vi "Apply Density.vi"(0 "ToneCloud in":refnum<class "Tone Cloud.lvclass">, 11 "error in (no error)":errorcluster) -> (4 "ToneCloud out":refnum<class "Tone Cloud.lvclass">, 15 "error out":errorcluster)   [LabVIEW 2015, in "Tone Cloud.lvclass"]
uses:
  Tone Cloud.lvclass
  Tone Cloud.lvclass/Tone Cloud.ctl
  <vilib>/regexp/Match Regular Expression.xnode
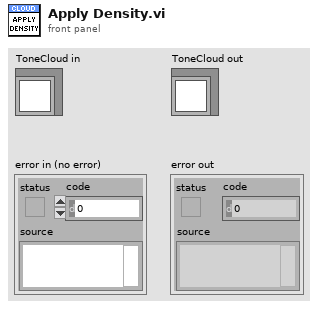
[diagram p1: front panel]
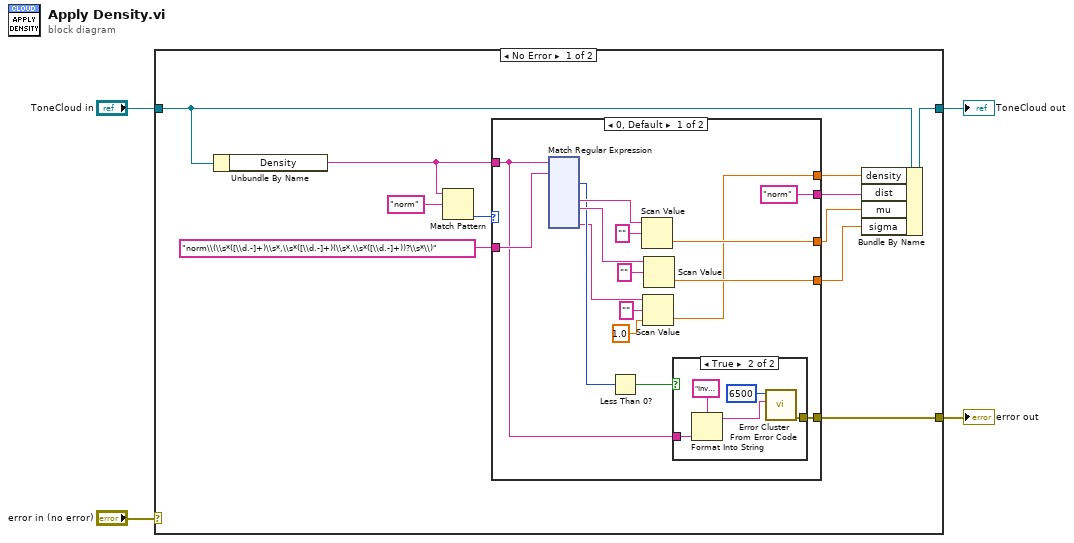
[diagram p0: block diagram]
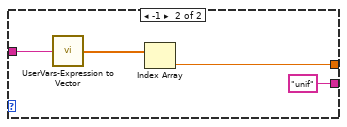
[diagram p3: hidden frame]
diagram:
  n1 = case shown="No Error" "error in (no error)" {
    selector: "error in (no error)" -> [_ w161]
    tunnel: [w5 w161] -> w3
    tunnel: [w14 w160] -> w1
    tunnel: "ToneCloud in" -> [w15 w160]
    frame No Error {
      n2 = Unbundle By Name(w15) -> ("Density"=w12:string)
      n3 = Match Pattern(string=w12, regular expression="norm") -> (offset past match=w10:i32)  [unwired: 1 in, 3 out]
      n4 = case shown="0, Default" w10 {
        tunnel: [w16 w158] -> w13
        tunnel: w12 -> [w21 w157]
        tunnel: ["norm" "unif"] -> w9
        tunnel: "norm\\(\\s*([\\d.-]+)\\s*,\\s*([\\d.-]+)(\\s*,\\s*([\\d.-]+))?\\s*\\)" ("String") -> [w30 _]
        tunnel: [w28 _] -> w7
        tunnel: [w24 _] -> w6
        tunnel: [w20 _] -> w5
        frame 0, Default {
          n5 = xnode "Match Regular Expression"("input string"=w21, "regular expression"=w30) -> ("offset past match"=w23:i32, "submatch 1"=w29:string, "submatch 2"=w25:string, "submatch 4"=w18:string)  [unwired: 4 in, 5 out]
          n6 = Less Than 0?(x=w23) -> (x < 0?=w22:bool)
          n7 = Scan Value(string=w29, format string="") -> (value=w28:dbl)  [unwired: 1 in, 1 out]
          n8 = Scan Value(string=w18, format string="", default (0 dbl)=1.0) -> (value=w16:dbl)  [unwired: 1 out]
          n9 = Scan Value(string=w25, format string="") -> (value=w24:dbl)  [unwired: 1 in, 1 out]
          n10 = case shown="True" w22 {
            tunnel: w21 -> [_ w152]
            tunnel: [_ w151] -> w20
            frame False {
            }
            frame True {
              n11 = Format Into String(format string="Invalid Tone Cloud density: '%s'", w152) -> (resulting string=w155:string)  [unwired: 2 in, 1 out]
              n12 = call <vilib>:"Error Cluster From Error Code.vi"("error message (\"\")"=w155, "error code (0)"=6500) -> ("error out"=w151:errorcluster)  [unwired: 7 in]
            }
          }
        }
        frame -1 {
          n13 = call "UserVars-Expression to Vector.vi"("Expr"=w157) -> ("Values"=w159:dbl[])  [unwired: 13 in, 1 out]
          n14 = Index Array(array=w159) -> (element=w158:dbl)  [unwired: 1 in]
        }
      }
      n15 = Bundle By Name(cluster=w15, "density"=w13, "dist"=w9, "mu"=w7, "sigma"=w6) -> (w14:refnum<class "Tone Cloud.lvclass">)
    }
    frame Error {
    }
  }
  "error out" <- w3
  "ToneCloud out" <- w1
